vi "Set Assistance.vi"(8 "error in":errorcluster, 11 "assistance?":bool) -> (0 "error out":errorcluster)   [LabVIEW 2017, in "myPAM.lvlib"]
uses:
  myPAM.lvlib
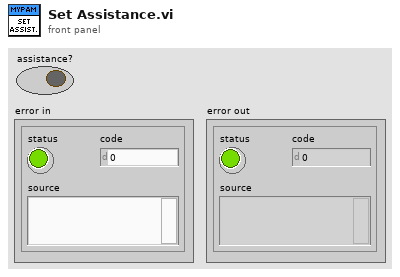
[diagram p1: front panel]
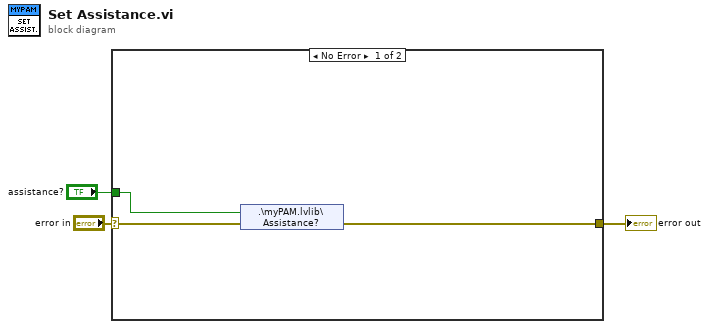
[diagram p0: block diagram]
diagram:
  n1 = case shown="No Error" "error in" {
    selector: "error in" -> [w6 w7]
    tunnel: [w5 w7] -> w3
    tunnel: "assistance?" -> [w4 _]
    frame No Error {
      n2 = shared-variable ".\\myPAM.lvlib\\Assistance?"(w4, error in=w6) -> (error out=w5:errorcluster)
    }
    frame Error {
    }
  }
  "error out" <- w3
